vi "savespectramonocoup_SD.vi"(0 "Data":dbl[][](array[numeric]), 1 "nom":string, 2 "chemin du dossier":path, 3 "String":string) -> ()   [LabVIEW 2015]
uses:
  <vilib>/Utility/file.llb/Write To Spreadsheet File (DBL).vi
  globalVarSD.vi
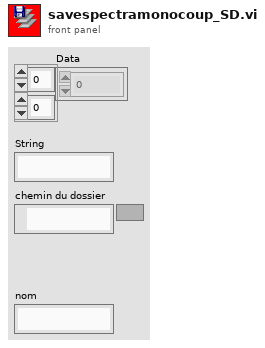
[diagram p1: front panel]
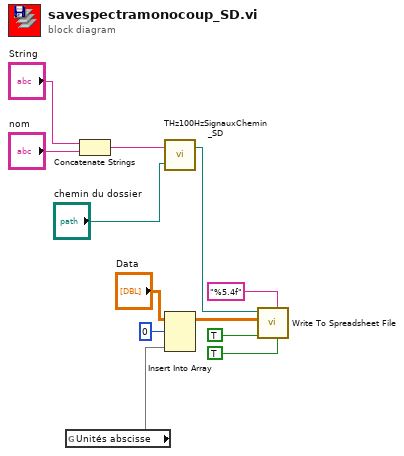
[diagram p0: block diagram]
diagram:
  n1 = global read "globalVarSD.vi" "Unités abscisse"() -> (w1)
  n2 = Concatenate Strings("String", "nom") -> (w5:string)
  n3 = call "THz100HzSignauxChemin_SD.vi"("chemin du dossier"="chemin du dossier", "nom"=w5) -> ("chemin du fichier DAT"=w4:path)  [unwired: 1 out]
  n4 = Insert Into Array(array="Data", index (row)=0 ("indice (ligne)"), new element=w1) -> (w3:dbl[][])  [unwired: 1 in]
  n5 = call-poly <vilib>:"Write To Spreadsheet File.vi"("transpose? (no:F)"=TRUE, "format (%.3f)"="%5.4f", "append to file? (new file:F)"=TRUE, "2D data"=w3, "file path (dialog if empty)"=w4) -> ()  [unwired: 3 in, 1 out]
